vi "PressureGauge.vi"(4 "Error In":errorcluster, 7 "Command":string) -> (0 "Error Out":errorcluster, 3 "Response":string)   [LabVIEW 2018]
uses:
  MOKO_LabViewLibrary/MokoLowLevel/MokoLowLovelControl/MLLC_Mode.ctl
  data/PressureGaugeInfo.ctl
panel:
  in  "Utility Name":string="PRESSURESTORE"
  in  "Error Code":i32=5475
  in  "UtilitySettings":T2={"Permanent data"={"Информация об образце"={"Тип"="Манометр", "Владелец"="Компания \"MOKO\"", "Номер клейма"="111222", "Пределы допускаемой погрешности "=0.05, "Производственный № прибора"="111222333", "Наименование СИ"="Манометр"}, "Информация о поверке"={"Место проведения поверки"="Планета земля", "Поверку провел"="Johnny Respect", "Номер заказа"="1", "Номер рабочего места"="1", "ДД"=21.0, "ММ"="Январь", "ГГГГ"=2022.0, "№ протокола"="G-111111", "№ манометра"=5555.0}, "Характеристики манометра"={"Максимум шкалы"=10.0, "1-ая точка"=2.0, "Единица измерения"="МПа", "Цена деления"=2.0, "Класс точности"="0,4", "Минимум шкалы"=2.0, "Количество точек"=0.0}, "Условия поверки"={"Температура воздуха"=22.0, "Влажность воздуха"=60.0, "Давление"=750.0}, "Драйвер"="Simulation", "Поверяемая точка"=0.0}, "Saved Data"=variant(cluster{"Информация об образце":cluster{"Тип":string, "Владелец":string, "Номер клейма":string, "Пределы допускаемой погрешности ":dbl, "Производственный № прибора":string, "Наименование СИ":string}, "Информация о поверке":cluster{"Место проведения поверки":string, "Поверку провел":string, "Номер заказа":string, "Номер рабочего места":string, "ДД":dbl, "ММ":string, "ГГГГ":dbl, "№ протокола":string, "№ манометра":dbl}, "Характеристики манометра":cluster{"Максимум шкалы":dbl, "1-ая точка":dbl, "Единица измерения":string, "Цена деления":dbl, "Класс точности":string, "Минимум шкалы":dbl, "Количество точек":dbl}, "Условия поверки":cluster{"Температура воздуха":dbl, "Влажность воздуха":dbl, "Давление":dbl}, "Драйвер":string, "Поверяемая точка":dbl} {"Информация об образце"={"Тип"="Манометр", "Владелец"="Компания \"MOKO\"", "Номер клейма"="111222333", "Пределы допускаемой погрешности "=0.05, "Производственный № прибора"="111222333", "Наименование СИ"="Манометр"}, "Информация о поверке"={"Место проведения поверки"="Планета земля", "Поверку провел"="Johnny Respect", "Номер заказа"="1", "Номер рабочего места"="1", "ДД"=21.0, "ММ"="Январь", "ГГГГ"=2022.0, "№ протокола"="G-111111", "№ манометра"=1123123.0}, "Характеристики манометра"={"Максимум шкалы"=10.0, "1-ая точка"=2.0, "Единица измерения"="МПа", "Цена деления"=2.0, "Класс точности"="0,4", "Минимум шкалы"=2.0, "Количество точек"=0.0}, "Условия поверки"={"Температура воздуха"=22.0, "Влажность воздуха"=60.0, "Давление"=750.0}, "Драйвер"="Simulation", "Поверяемая точка"=0.0}), "waittime"=30000.0, "BAD"=0.0, "Defect"=FALSE}
  in  "Mode":T3=enum."Check"
  # "PressureGauge"
  # "Default Settings"
  # "Temporary data"
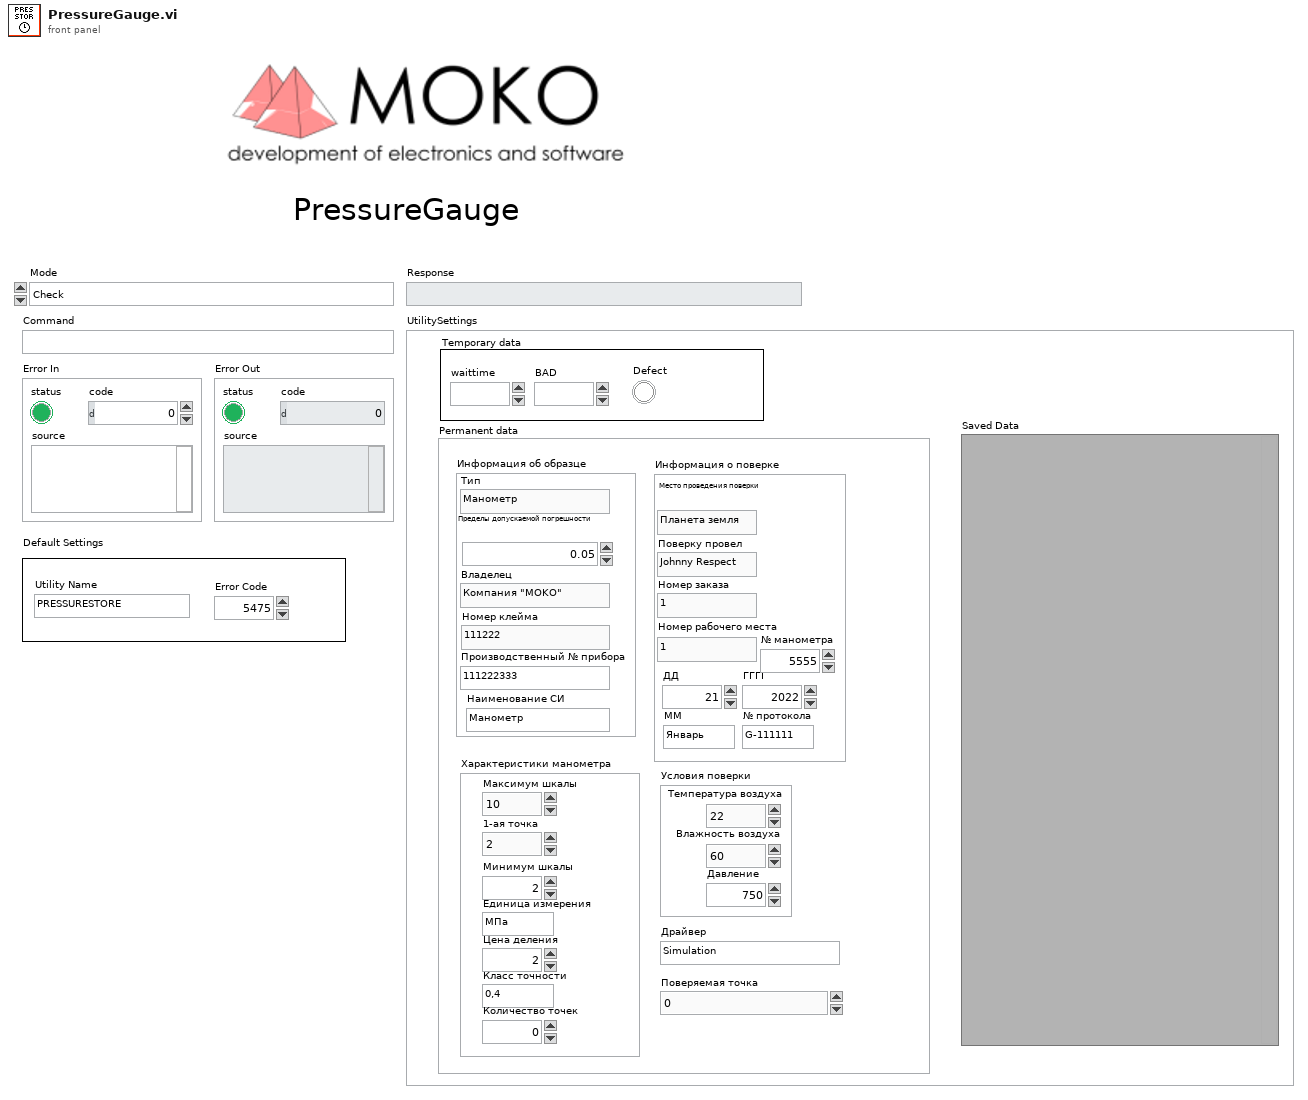
[diagram p1: front panel]
types:
  T1 = typedef "PressureGaugeInfo.ctl" = cluster{"Информация об образце":cluster{"Тип":string, "Владелец":string, "Номер клейма":string, "Пределы допускаемой погрешности ":dbl, "Производственный № прибора":string, "Наименование СИ":string}, "Информация о поверке":cluster{"Место проведения поверки":string, "Поверку провел":string, "Номер заказа":string, "Номер рабочего места":string, "ДД":dbl, "ММ":string, "ГГГГ":dbl, "№ протокола":string, "№ манометра":dbl}, "Характеристики манометра":cluster{"Максимум шкалы":dbl, "1-ая точка":dbl, "Единица измерения":string, "Цена деления":dbl, "Класс точности":string, "Минимум шкалы":dbl, "Количество точек":dbl}, "Условия поверки":cluster{"Температура воздуха":dbl, "Влажность воздуха":dbl, "Давление":dbl}, "Драйвер":string, "Поверяемая точка":dbl}
  T2 = cluster{"Permanent data":T1, "Saved Data":variant, "waittime":dbl, "BAD":dbl, "Defect":bool}
  T3 = typedef "MLLC_Mode.ctl" = enum16{"get", "set", "close", "Init", "Check"}
  T4 = typedef "MLLC_Error.ctl" = errorcluster
  T5 = typedef "MLLC_Command.ctl" = string
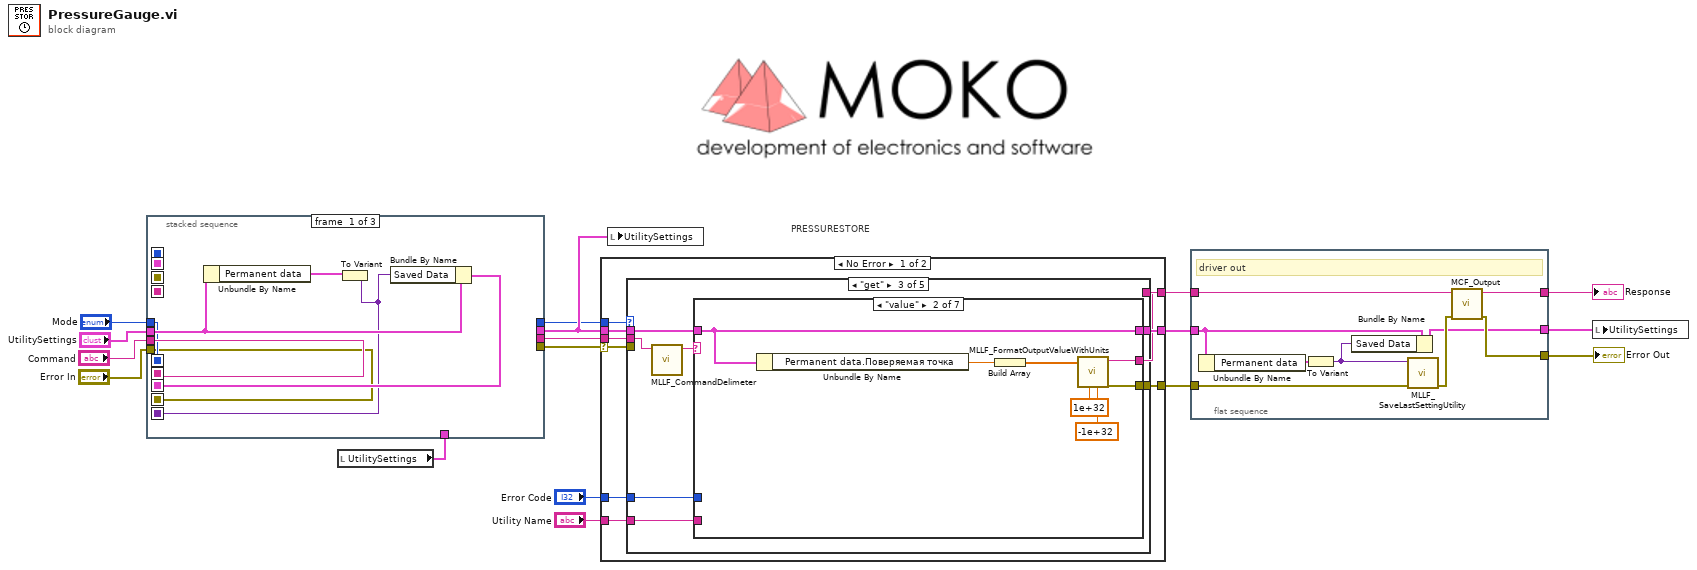
[diagram p0: block diagram]
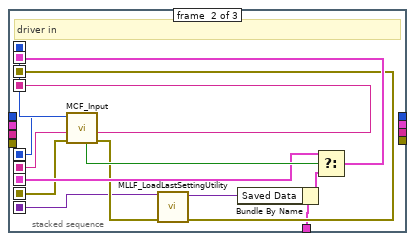
[diagram p2: hidden frame]
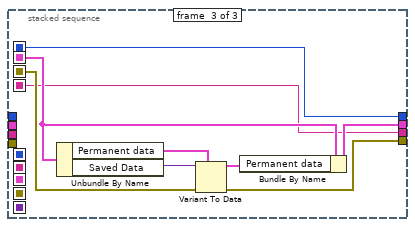
[diagram p3: hidden frame]
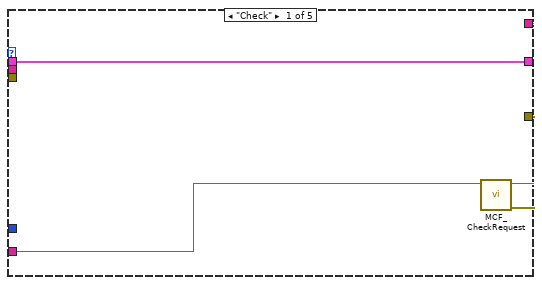
[diagram p4: hidden frame]
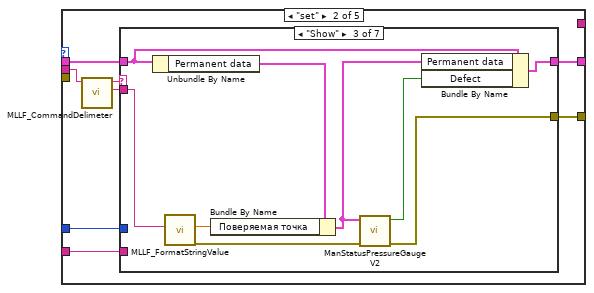
[diagram p5: hidden frame]
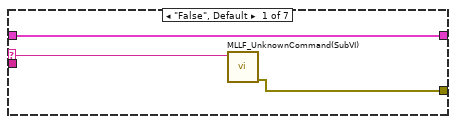
[diagram p6: hidden frame]
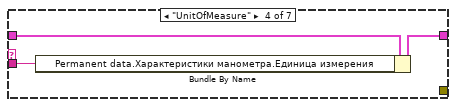
[diagram p8: hidden frame]
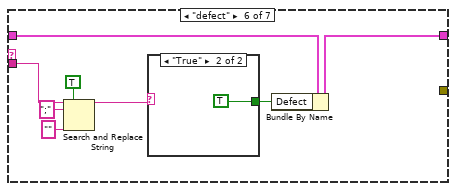
[diagram p10: hidden frame]
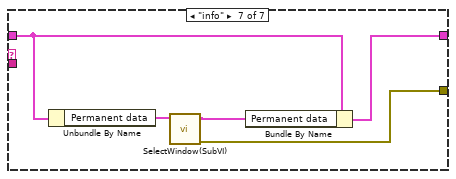
[diagram p12: hidden frame]
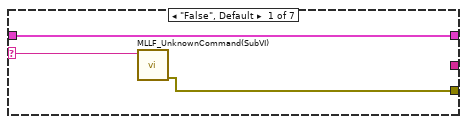
[diagram p13: hidden frame]
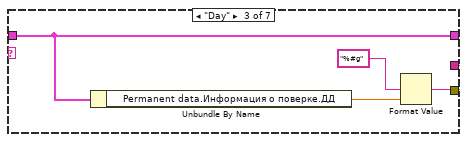
[diagram p14: hidden frame]
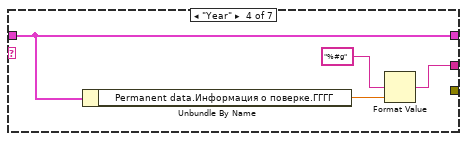
[diagram p15: hidden frame]
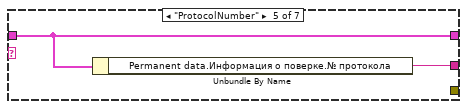
[diagram p16: hidden frame]
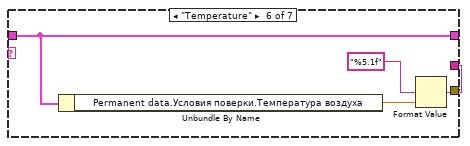
[diagram p17: hidden frame]
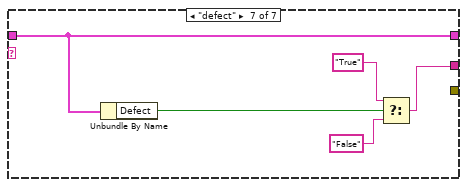
[diagram p18: hidden frame]
diagram:
  # "PRESSURESTORE"
  n1 = local read "UtilitySettings"() -> (w12:T2)
  n2 = stacked-sequence {
    seq-local: [w20 _ _] -> [_ w36 _]
    seq-local: [w19 _ _] -> [_ w37 _]
    seq-local: [w22 _ _] -> [_ w32 _]
    seq-local: [w18 _ _] -> [_ w31 _]
    seq-local: [w21 _ _] -> [_ w26 _]
    seq-local: [_ w27 _] -> [_ _ w43]
    seq-local: [_ w38 _] -> [_ _ w40]
    seq-local: [_ w35 _] -> [_ _ w39]
    seq-local: [_ w34 _] -> [_ _ w44]
    tunnel: "Command" -> [w20 _ _]
    tunnel: "Mode" -> [w19 _ _]
    tunnel: "Error In" -> [w18 _ _]
    tunnel: "UtilitySettings" -> [w23 _ _]
    tunnel: w12 -> [_ w25 _]
    tunnel: [_ _ w39] -> w8
    tunnel: [_ _ w42] -> w11
    tunnel: [_ _ w41] -> w10
    tunnel: [_ _ w40] -> w9
    frame #0 {
      n3 = Unbundle By Name(w23) -> ("Permanent data"=w24:T1)
      n4 = To Variant(anything=w24) -> (Variant=w21:variant)
      n5 = Bundle By Name(cluster=w23, "Saved Data"=w21) -> (w22:T2)
    }
    frame #1 {
      # "driver in"
      n6 = call "MCF_Input.vi"("error in (no error)"=w31, "Command"=w36, "Mode"=w37) -> ("error out"=w30:errorcluster, "Command out"=w35:string, "Mode out"=w38:T3, "Boolean"=w33:bool)  [unwired: 5 in]
      n7 = call "MLLF_LoadLastSettingUtility.vi"("Error In"=w30, "Save data in"=w26) -> ("Error Out"=w27:errorcluster, "Save data out"=w29:variant)  [unwired: 8 in]
      n8 = Bundle By Name(cluster=w25, "Saved Data"=w29) -> (w28:T2)
      n9 = Select(t=w32, s=w33, f=w28) -> (s? t:f=w34:T2)
    }
    frame #2 {
      n10 = Unbundle By Name(w44) -> ("Permanent data"=w45:T1, "Saved Data"=w47:variant)
      n11 = Variant To Data(error in=w43, type=w45, Variant=w47) -> (data=w46:T1, error out=w41:errorcluster)
      n12 = Bundle By Name(cluster=w44, "Permanent data"=w46) -> (w42:T2)
    }
  }
  n13 = case shown="No Error" w10 {
    selector: w10 -> [w52 w138]
    tunnel: [w54 w138] -> w16
    tunnel: w9 -> [w56 _]
    tunnel: [w55 _] -> w14
    tunnel: w8 -> [w53 _]
    tunnel: w11 -> [w49 w137]
    tunnel: "Error Code" -> [w51 _]
    tunnel: "Utility Name" -> [w50 _]
    tunnel: [w48 w137] -> w15
    frame No Error {
      n14 = case shown="\"get\"" w56 {
        tunnel: [w58 _ w100 _ _] -> w55
        tunnel: [w57 w62 w101 _ _] -> w54
        tunnel: w53 -> [_ w68 w107 _ _]
        tunnel: w52 -> [_ _ _ _ _]
        tunnel: w51 -> [_ w67 w104 _ _]
        tunnel: w50 -> [w59 w64 w103 _ _]
        tunnel: w49 -> [w60 w66 w106 _ _]
        tunnel: [w60 w65 w105 _ _] -> w48
        frame "Check" {
          n15 = call "MCF_CheckRequest.vi"("Driver Name"=w59) -> ("Error Out"=w57:errorcluster, "Output String"=w58:string)  [unwired: 9 in]
        }
        frame "set" {
          n16 = call "MLLF_CommandDelimeter.vi"("command with param"=w68) -> ("param 1"=w61:string, "command"=w63:string)  [unwired: 7 in, 2 out]
          n17 = case shown="\"Show\"" w63 {
            selector: w63 -> [w70 _ _ _ _ _ _]
            tunnel: w61 -> [_ _ w78 w83 _ w91 _]
            tunnel: [w69 _ w75 _ _ _ w95] -> w62
            tunnel: w67 -> [_ _ _ _ _ _ _]
            tunnel: w66 -> [w71 w72 w80 w84 w85 w93 w99]
            tunnel: [w71 w72 w79 w82 w85 w92 w98] -> w65
            tunnel: w64 -> [_ _ _ _ _ _ _]
            frame "False", Default {
              n18 = call "MLLF_UnknownCommand(SubVI).vi"("Unknown command"=w70) -> ("error out"=w69:errorcluster)  [unwired: 10 in]
            }
            frame "<----MAIN FUNCTIONS---->" {
            }
            frame "Show" {
              n19 = Unbundle By Name(w80) -> ("Permanent data"=w74:T1)
              n20 = call "MLLF_FormatStringValue.vi"("String Value"=w78) -> ("error out"=w77:T4, "number"=w81:dbl)  [unwired: 8 in, 1 out]
              n21 = Bundle By Name(cluster=w74, "Поверяемая точка"=w81) -> (w73:T1)
              n22 = call "ManStatusPressureGaugeV2.vi"("Error In"=w77, "Show in"=w73) -> ("Error Out"=w75:errorcluster, "defect"=w76:bool)  [unwired: 8 in]
              n23 = Bundle By Name(cluster=w80, "Permanent data"=w73, "Defect"=w76) -> (w79:T2)
            }
            frame "UnitOfMeasure" {
              n24 = Bundle By Name(cluster=w84, "Permanent data.Характеристики манометра.Единица измерения"=w83) -> (w82:T2)
            }
            frame "---------ADDITIONAL---------" {
            }
            frame "defect" {
              n25 = Search and Replace String(replace all?=TRUE ("replace all? (F)"), input string=w91, search string=";", replace string="" ("replace string (\"\")")) -> (result string=w87:string)  [unwired: 4 in, 3 out]
              n26 = case shown="\"True\"" w87 {
                tunnel: [_ TRUE] -> w86
                frame "False", Default {
                }
                frame "True" {
                }
              }
              n27 = Bundle By Name(cluster=w93, "Defect"=w86) -> (w92:T2)
            }
            frame "info" {
              n28 = Unbundle By Name(w99) -> ("Permanent data"=w97:T1)
              n29 = call "SelectWindow(SubVI).vi"("Permanent data"=w97) -> ("Error Out"=w95:errorcluster, "Manometr out"=w96:T1)  [unwired: 9 in]
              n30 = Bundle By Name(cluster=w99, "Permanent data"=w96) -> (w98:T2)
            }
          }
        }
        frame "get" {
          n31 = call "MLLF_CommandDelimeter.vi"("command with param"=w107) -> ("command"=w102:string)  [unwired: 7 in, 3 out]
          n32 = case shown="\"value\"" w102 {
            selector: w102 -> [w109 _ _ _ _ _ _]
            tunnel: [w108 w111 _ _ _ _ _] -> w101
            tunnel: w104 -> [_ _ _ _ _ _ _]
            tunnel: [w110 w117 w121 w125 w127 w131 w136] -> w105
            tunnel: w106 -> [w110 w117 w121 w125 w127 w131 w136]
            tunnel: w103 -> [_ _ _ _ _ _ _]
            tunnel: [_ w112 w118 w122 w126 w128 w132] -> w100
            frame "False", Default {
              n33 = call "MLLF_UnknownCommand(SubVI).vi"("Unknown command"=w109) -> ("error out"=w108:errorcluster)  [unwired: 10 in]
            }
            frame "value" {
              n34 = Unbundle By Name(w117) -> ("Permanent data.Поверяемая точка"=w116:dbl)
              n35 = Build Array(w116) -> (w113:dbl[])
              n36 = call "MLLF_FormatOutputValueWithUnits.vi"("Lower limit"=-1e+32, "Upper limit"=1e+32, "ValuesIn"=w113) -> ("error out"=w111:T4, "Result string"=w112:T5)  [unwired: 7 in]
            }
            frame "Day" {
              n37 = Unbundle By Name(w121) -> ("Permanent data.Информация о поверке.ДД"=w119:dbl)
              n38 = Format Value(format string="%#g", value (0)=w119) -> (output string=w118:string)  [unwired: 1 in]
            }
            frame "Year" {
              n39 = Unbundle By Name(w125) -> ("Permanent data.Информация о поверке.ГГГГ"=w123:dbl)
              n40 = Format Value(format string="%#g", value (0)=w123) -> (output string=w122:string)  [unwired: 1 in]
            }
            frame "ProtocolNumber" {
              n41 = Unbundle By Name(w127) -> ("Permanent data.Информация о поверке.№ протокола"=w126:string)
            }
            frame "Temperature" {
              n42 = Unbundle By Name(w131) -> ("Permanent data.Условия поверки.Температура воздуха"=w130:dbl)
              n43 = Format Value(format string="%5.1f", value (0)=w130) -> (output string=w128:string)  [unwired: 1 in]
            }
            frame "defect" {
              n44 = Unbundle By Name(w136) -> ("Defect"=w133:bool)
              n45 = Select(t="True" ("string"), s=w133, f="False" ("string")) -> (s? t:f=w132:string)
            }
          }
        }
        frame "close" {
        }
        frame "Init" {
        }
      }
    }
    frame Error {
    }
  }
  n46 = local write "UtilitySettings"(w11) -> ()
  n47 = flat-sequence {
    tunnel: [w147] -> w6
    tunnel: [w146] -> w4
    tunnel: w14 -> [w145]
    tunnel: w16 -> [w144]
    tunnel: w15 -> [w140]
    tunnel: [w142] -> w13
    frame #0 {
      # "driver out"
      n48 = Unbundle By Name(w140) -> ("Permanent data"=w139:T1)
      n49 = To Variant(anything=w139) -> (Variant=w141:variant)
      n50 = Bundle By Name(cluster=w140, "Saved Data"=w141) -> (w142:T2)
      n51 = call "MLLF_SaveLastSettingUtility.vi"("error in"=w144, "Saved Data"=w141) -> ("error out"=w143:T4)  [unwired: 8 in, 1 out]
      n52 = call "MCF_Output.vi"("Error In"=w143, "Input"=w145) -> ("Error Out"=w146:errorcluster, "Output"=w147:string)  [unwired: 8 in]
    }
  }
  n53 = local write "UtilitySettings"(w13) -> ()
  "Response" <- w6
  "Error Out" <- w4
